vi "Update Test Results.vi"(6 "Positions":i32[](array[numeric]), 8 "error in (no error)":errorcluster, 9 "Tests Passed":bool[](array[boolean]), 10 "Fail Codes":string[](array[string]), 11 "Application in":refnum<class "Application.lvclass">) -> (0 "error out":errorcluster, 3 "Application in":refnum<class "Application.lvclass">)   [LabVIEW 2017, in "Application.lvlib" / "Application.lvclass"]
doc: "Used after a test has run to update the pass/fail status for each position, as well as add fail codes to the fail code string."
uses:
  Application.lvclass
  Application.lvclass/Application.ctl
  Properties/App Properties.lvclass
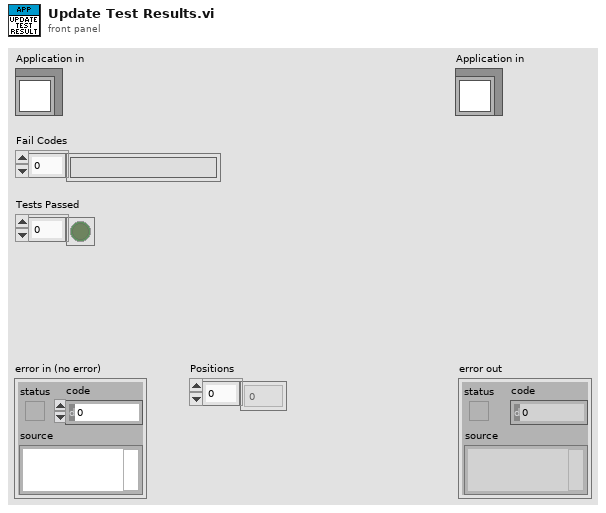
[diagram p1: front panel]
types:
  T1 = typedef "Application.lvlib/App Properties.lvclass/Class Properties -- Cluster.ctl" = cluster{"UUT Info":T2[], "Test Information":refnum<vi>, "Gold Board":refnum<class "Golden Board.lvclass">, "Test Recipe":refnum<class "Test Recipe.lvclass">, "Instruments":refnum<class "Instrument.lvclass">[], "Mode":T3, "Test Results":T4[], "Station Config":refnum<class "Station Config.lvclass">, "Variable Engine":refnum<class "Variable Engine.lvclass">}
  T2 = typedef "Application.lvlib/App Properties.lvclass/UUT Reference -- Cluster.ctl" = cluster{"Serial Number Reference":refnum<vi>, "Status Message Reference":refnum<vi>}
  T3 = typedef "Application.lvlib/Application.lvclass/Op Mode -- Enum.ctl" = u16
  T4 = typedef "Application.lvlib/App Properties.lvclass/Test Result -- Cluster.ctl" = cluster{"Position":i32, "Pass":bool, "Fail Codes":string}
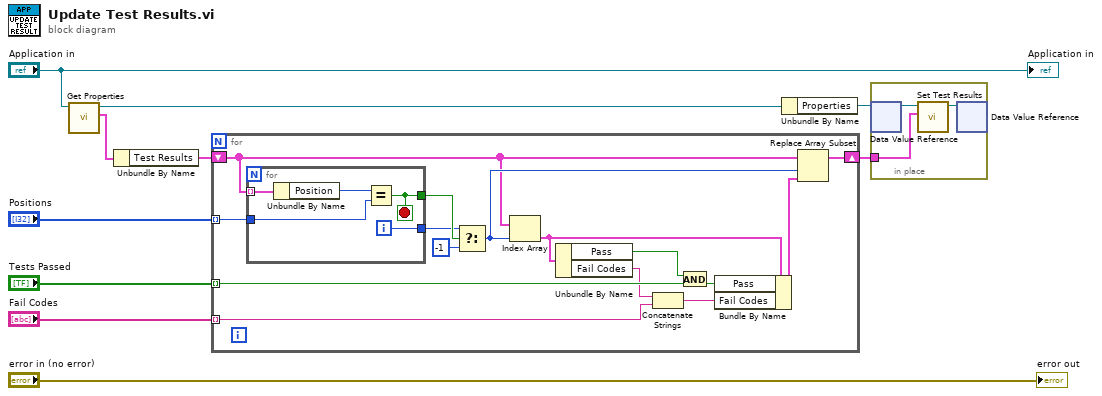
[diagram p0: block diagram]
diagram:
  n1 = call "Get Properties.vi"("Acrobat Template in"="Application in") -> ("Class Properties"=w6:T1, "Acrobat Template out"=w4:refnum<class "Application.lvclass">)  [unwired: 8 in, 1 out]
  n2 = Unbundle By Name(w6) -> ("Test Results"=w5:T4[])
  n3 = for {
    tunnel: "Positions" -> [w22] mode=indexing
    tunnel: "Tests Passed" -> [w15] mode=indexing
    tunnel: "Fail Codes" -> [w12] mode=indexing
    shift-right: [w20] -> w2
    shift-left: w5 -> [w11]
    n4 = for {
      tunnel: w11 -> [w30] mode=indexing
      tunnel: w22 -> [w28]
      tunnel: [w27] -> w23
      tunnel: [w26] -> w24
      i -> [w27]
      stop <- w26 stop-if-true
      n5 = Unbundle By Name(w30) -> ("Position"=w29:i32)
      n6 = Equal?(x=w29, y=w28) -> (x = y?=w26:bool)
    }
    n7 = Select(t=w23, s=w24, f=-1) -> (s? t:f=w19:i32)
    n8 = Index Array(array=w11, index=w19) -> (element=w18:T4)
    n9 = Unbundle By Name(w18) -> ("Pass"=w17:bool, "Fail Codes"=w13:string)
    n10 = Concatenate Strings(w13, w12) -> (w14:string)
    n11 = And(x=w17, y=w15) -> (x .and. y?=w16:bool)
    n12 = Bundle By Name(cluster=w18, "Pass"=w16, "Fail Codes"=w14) -> (w21:T4)
    n13 = Replace Array Subset(array=w11, new element=w21, index=w19) -> (w20:T4[])
  }
  n14 = Unbundle By Name(w4) -> ("Properties"=w3:refnum<data-value>)
  n15 = in-place {
    in-place-border: w2 -> [w33]
    n16 = in-place-dvr #1(w3) -> (w32:refnum<class "App Properties.lvclass">)  [unwired: 1 out]
    n17 = call-dynamic "Set Test Results.vi"("Test Results"=w33, "App Properties in"=w32) -> ("App Properties out"=w31:refnum<class "App Properties.lvclass">)  [unwired: 8 in, 1 out]
    n18 = in-place-dvr #1(w31) -> ()  [unwired: 2 out]
  }
  "error out" <- "error in (no error)"
  "Application in" <- "Application in"
